vi "Mod_OFDM_Examine_Configure_OFDM_Frame.vi"(0 "Configuration in":variant=variant("Attribute Names"=variant(cluster{"Data Source Pool":string, "Modulator Source Pool":string, "OFDM SYMBOL POOL":string, "Symbol Table":string, "Sub Carrier Selection":string, "OFDM Frame":string, "FRAME Table":string, "Pulse Shaping":string} {"Data Source Pool"="Data Source ", "Modulator Source Pool"="Modulator Source Pool ", "OFDM SYMBOL POOL"="OFDM SYMBOL POOL", "Symbol Table"="Symbol Table", "Sub Carrier Selection"="Sub Carrier Selection", "OFDM Frame"="OFDM Frame", "FRAME Table"="FRAME Table", "Pulse Shaping"="Pulse Shaping"}), "Data Source "=variant(cluster{"mode (PN)":enum16{"PN", "pattern", "user"}, "PN sequence order (9)":i32, "Invert Output Bits":enum16{"No", "Yes"}, "Register Initial State":u32, "User base bit pattern":i8[], "base bit pattern (00001111)":enum16{"0", "1", "01", "0011", "00001111"}, "Reset to Initial State":enum16{"Every OFDM Frame", "Every OFDM Symbol", "Every Sub Carrier"}}[] [{"mode (PN)"=enum."PN", "PN sequence order (9)"=9, "Invert Output Bits"=enum."No", "Register Initial State"=3602873842, "User base bit pattern"=[], "base bit pattern (00001111)"=enum."00001111", "Reset to Initial State"=enum."Every OFDM Frame"}, {"mode (PN)"=enum."PN", "PN sequence order (9)"=9, "Invert Output Bits"=enum."No", "Register Initial State"=3602873842, "User base bit pattern"=[], "base bit pattern (00001111)"=enum."00001111", "Reset to Initial State"=enum."Every OFDM Frame"}, {"mode (PN)"=enum."PN", "PN sequence order (9)"=9, "Invert Output Bits"=enum."No", "Register Initial State"=3602873842, "User base bit pattern"=[], "base bit pattern (00001111)"=enum."00001111", "Reset to Initial State"=enum."Every OFDM Frame"}, {"mode (PN)"=enum."PN", "PN sequence order (9)"=9, "Invert Output Bits"=enum."No", "Register Initial State"=3602873842, "User base bit pattern"=[], "base bit pattern (00001111)"=enum."00001111", "Reset to Initial State"=enum."Every OFDM Frame"}]), "FRAME Table"=variant(string[][] []), "Modulator Source Pool "=variant(cluster{"M-QAM":enum16{"4", "16", "64", "256"}, "M-PSK":enum16{"2", "4", "8", "16", "32", "64", "128", "256"}, "Type of Modulation":enum16{"PSK", "QAM"}, "PSK":cluster{"differential PSK":enum16{"disable", "enable"}, "PSK type":enum16{"normal", "shifted", "offset"}}}[] [{"M-QAM"=enum."4", "M-PSK"=enum."2", "Type of Modulation"=enum."PSK", "PSK"={"differential PSK"=enum."disable", "PSK type"=enum."normal"}}, {"M-QAM"=enum."4", "M-PSK"=enum."2", "Type of Modulation"=enum."PSK", "PSK"={"differential PSK"=enum."disable", "PSK type"=enum."normal"}}, {"M-QAM"=enum."4", "M-PSK"=enum."2", "Type of Modulation"=enum."PSK", "PSK"={"differential PSK"=enum."disable", "PSK type"=enum."normal"}}, {"M-QAM"=enum."4", "M-PSK"=enum."2", "Type of Modulation"=enum."PSK", "PSK"={"differential PSK"=enum."disable", "PSK type"=enum."normal"}}]), "No_Name"=variant(cluster{"Sub Carrier Selection":cluster{"Sub Carrier":bool, "Data Source":u16, "Modulator":u16}[], "OFDM Parameters":cluster{"# of Sub Carrier":i32, "Length Of Cylic Prefix":i32}} {"Sub Carrier Selection"=[{"Sub Carrier"=TRUE, "Data Source"=0, "Modulator"=0}, {"Sub Carrier"=TRUE, "Data Source"=0, "Modulator"=0}, {"Sub Carrier"=TRUE, "Data Source"=0, "Modulator"=0}, {"Sub Carrier"=TRUE, "Data Source"=0, "Modulator"=0}, {"Sub Carrier"=TRUE, "Data Source"=0, "Modulator"=0}, {"Sub Carrier"=TRUE, "Data Source"=0, "Modulator"=0}, {"Sub Carrier"=TRUE, "Data Source"=0, "Modulator"=0}, {"Sub Carrier"=TRUE, "Data Source"=0, "Modulator"=0}, {"Sub Carrier"=TRUE, "Data Source"=0, "Modulator"=0}, {"Sub Carrier"=TRUE, "Data Source"=0, "Modulator"=0}, {"Sub Carrier"=TRUE, "Data Source"=0, "Modulator"=0}, {"Sub Carrier"=TRUE, "Data Source"=0, "Modulator"=0}, {"Sub Carrier"=TRUE, "Data Source"=0, "Modulator"=0}, {"Sub Carrier"=TRUE, "Data Source"=0, "Modulator"=0}, {"Sub Carrier"=TRUE, "Data Source"=0, "Modulator"=0}, {"Sub Carrier"=TRUE, "Data Source"=0, "Modulator"=0}, {"Sub Carrier"=TRUE, "Data Source"=0, "Modulator"=0}, {"Sub Carrier"=TRUE, "Data Source"=0, "Modulator"=0}, {"Sub Carrier"=TRUE, "Data Source"=0, "Modulator"=0}, {"Sub Carrier"=TRUE, "Data Source"=0, "Modulator"=0}, {"Sub Carrier"=TRUE, "Data Source"=0, "Modulator"=0}, {"Sub Carrier"=TRUE, "Data Source"=0, "Modulator"=0}, {"Sub Carrier"=TRUE, "Data Source"=0, "Modulator"=0}, {"Sub Carrier"=TRUE, "Data Source"=0, "Modulator"=0}, {"Sub Carrier"=TRUE, "Data Source"=0, "Modulator"=0}, {"Sub Carrier"=TRUE, "Data Source"=0, "Modulator"=0}, {"Sub Carrier"=TRUE, "Data Source"=0, "Modulator"=0}, {"Sub Carrier"=TRUE, "Data Source"=0, "Modulator"=0}, {"Sub Carrier"=TRUE, "Data Source"=0, "Modulator"=0}, {"Sub Carrier"=TRUE, "Data Source"=0, "Modulator"=0}, {"Sub Carrier"=TRUE, "Data Source"=0, "Modulator"=0}, {"Sub Carrier"=TRUE, "Data Source"=0, "Modulator"=0}, {"Sub Carrier"=TRUE, "Data Source"=0, "Modulator"=0}, {"Sub Carrier"=TRUE, "Data Source"=0, "Modulator"=0}, {"Sub Carrier"=TRUE, "Data Source"=0, "Modulator"=0}, {"Sub Carrier"=TRUE, "Data Source"=0, "Modulator"=0}, {"Sub Carrier"=TRUE, "Data Source"=0, "Modulator"=0}, {"Sub Carrier"=TRUE, "Data Source"=0, "Modulator"=0}, {"Sub Carrier"=TRUE, "Data Source"=0, "Modulator"=0}, {"Sub Carrier"=TRUE, "Data Source"=0, "Modulator"=0}, {"Sub Carrier"=TRUE, "Data Source"=0, "Modulator"=0}, {"Sub Carrier"=TRUE, "Data Source"=0, "Modulator"=0}, {"Sub Carrier"=TRUE, "Data Source"=0, "Modulator"=0}, {"Sub Carrier"=TRUE, "Data Source"=0, "Modulator"=0}, {"Sub Carrier"=TRUE, "Data Source"=0, "Modulator"=0}, {"Sub Carrier"=TRUE, "Data Source"=0, "Modulator"=0}, {"Sub Carrier"=TRUE, "Data Source"=0, "Modulator"=0}, {"Sub Carrier"=TRUE, "Data Source"=0, "Modulator"=2}, {"Sub Carrier"=TRUE, "Data Source"=0, "Modulator"=0}, {"Sub Carrier"=TRUE, "Data Source"=0, "Modulator"=0}, {"Sub Carrier"=TRUE, "Data Source"=0, "Modulator"=0}, {"Sub Carrier"=TRUE, "Data Source"=0, "Modulator"=0}, {"Sub Carrier"=TRUE, "Data Source"=0, "Modulator"=0}, {"Sub Carrier"=TRUE, "Data Source"=0, "Modulator"=0}, {"Sub Carrier"=TRUE, "Data Source"=0, "Modulator"=0}, {"Sub Carrier"=TRUE, "Data Source"=0, "Modulator"=0}, {"Sub Carrier"=TRUE, "Data Source"=0, "Modulator"=0}, {"Sub Carrier"=TRUE, "Data Source"=0, "Modulator"=0}, {"Sub Carrier"=TRUE, "Data Source"=0, "Modulator"=0}, {"Sub Carrier"=TRUE, "Data Source"=0, "Modulator"=0}, {"Sub Carrier"=TRUE, "Data Source"=0, "Modulator"=0}, {"Sub Carrier"=TRUE, "Data Source"=0, "Modulator"=0}, {"Sub Carrier"=TRUE, "Data Source"=0, "Modulator"=0}, {"Sub Carrier"=TRUE, "Data Source"=0, "Modulator"=0}], "OFDM Parameters"={"# of Sub Carrier"=64, "Length Of Cylic Prefix"=16}}), "OFDM Frame"=variant(cluster{"Symbol Name":string, "# of Symbols":i32}[] []), "OFDM SYMBOL POOL"=variant(string[] ["No_Name"]), "Pulse Shaping"=variant(cluster{"System Filter":cluster{"TX Filter":enum16{"none", "Raised Cosine", "Root Raised Cos"}, "Alpha":dbl, "filter length":i32}, "Modulation system parameters":cluster{"samples per symbol (16)":u32}, "symbol rate (Hz)":dbl} {"System Filter"={"TX Filter"=enum."Root Raised Cos", "Alpha"=0.5, "filter length"=8}, "Modulation system parameters"={"samples per symbol (16)"=16}, "symbol rate (Hz)"=100000.0}), "Sub Carrier Selection"=variant(cluster{"Sub Carrier Selection":cluster{"Sub Carrier":bool, "Data Source":u16, "Modulator":u16}[], "OFDM Parameters":cluster{"# of Sub Carrier":i32, "Length Of Cylic Prefix":i32}} {"Sub Carrier Selection"=array[10000 elements], "OFDM Parameters"={"# of Sub Carrier"=64, "Length Of Cylic Prefix"=16}}), "Symbol Table"=variant(string[][] [["-32", " ON", "   0", "   0"], ["-31", " ON", "   0", "   0"], ["-30", " ON", "   0", "   0"], ["-29", " ON", "   0", "   0"], ["-28", " ON", "   0", "   0"], ["-27", " ON", "   0", "   0"], ["-26", " ON", "   0", "   0"], ["-25", " ON", "   0", "   0"], ["-24", " ON", "   0", "   0"], ["-23", " ON", "   0", "   0"], ["-22", " ON", "   0", "   0"], ["-21", " ON", "   0", "   0"], ["-20", " ON", "   0", "   0"], ["-19", " ON", "   0", "   0"], ["-18", " ON", "   0", "   0"], ["-17", " ON", "   0", "   0"], ["-16", " ON", "   0", "   0"], ["-15", " ON", "   0", "   0"], ["-14", " ON", "   0", "   0"], ["-13", " ON", "   0", "   0"], ["-12", " ON", "   0", "   0"], ["-11", " ON", "   0", "   0"], ["-10", " ON", "   0", "   0"], ["-9", " ON", "   0", "   0"], ["-8", " ON", "   0", "   0"], ["-7", " ON", "   0", "   0"], ["-6", " ON", "   0", "   0"], ["-5", " ON", "   0", "   0"], ["-4", " ON", "   0", "   0"], ["-3", " ON", "   0", "   0"], ["-2", " ON", "   0", "   0"], ["-1", " ON", "   0", "   0"], ["0", " ON", "   0", "   0"], ["+1", " ON", "   0", "   0"], ["+2", " ON", "   0", "   0"], ["+3", " ON", "   0", "   0"], ["+4", " ON", "   0", "   0"], ["+5", " ON", "   0", "   0"], ["+6", " ON", "   0", "   0"], ["+7", " ON", "   0", "   0"], ["+8", " ON", "   0", "   0"], ["+9", " ON", "   0", "   0"], ["+10", " ON", "   0", "   0"], ["+11", " ON", "   0", "   0"], ["+12", " ON", "   0", "   0"], ["+13", " ON", "   0", "   0"], ["+14", " ON", "   0", "   0"], ["+15", " ON", "   0", "   2"], ["+16", " ON", "   0", "   0"], ["+17", " ON", "   0", "   0"], ["+18", " ON", "   0", "   0"], ["+19", " ON", "   0", "   0"], ["+20", " ON", "   0", "   0"], ["+21", " ON", "   0", "   0"], ["+22", " ON", "   0", "   0"], ["+23", " ON", "   0", "   0"], ["+24", " ON", "   0", "   0"], ["+25", " ON", "   0", "   0"], ["+26", " ON", "   0", "   0"], ["+27", " ON", "   0", "   0"], ["+28", " ON", "   0", "   0"], ["+29", " ON", "   0", "   0"], ["+30", " ON", "   0", "   0"], ["+31", " ON", "   0", "   0"]])), 5 "Configure OFDM Frame":T1={"Symbol Pool"=0, "Add"=FALSE, "Delete"=FALSE, "# of Symbols"=1} {"# of Symbols" min=1; "Symbol Pool" items=["IEEE 802.11a First Symbol of Frame", "IEEE 802.11a Frame (BPSK)", "IEEE 802.11a Frame (QPSK)", "IEEE 802.11a Frame (16QAM)", "IEEE 802.11a Frame (64QAM)", "No_Name"]}, 11 "error in":errorcluster) -> (4 "Configuration out":variant=variant("Attribute Names"=variant(cluster{"Data Source Pool":string, "Modulator Source Pool":string, "OFDM SYMBOL POOL":string, "Symbol Table":string, "Sub Carrier Selection":string, "OFDM Frame":string, "FRAME Table":string, "Pulse Shaping":string} {"Data Source Pool"="Data Source ", "Modulator Source Pool"="Modulator Source Pool ", "OFDM SYMBOL POOL"="OFDM SYMBOL POOL", "Symbol Table"="Symbol Table", "Sub Carrier Selection"="Sub Carrier Selection", "OFDM Frame"="OFDM Frame", "FRAME Table"="FRAME Table", "Pulse Shaping"="Pulse Shaping"}), "Data Source "=variant(cluster{"mode (PN)":enum16{"PN", "pattern", "user"}, "PN sequence order (9)":i32, "Invert Output Bits":enum16{"No", "Yes"}, "Register Initial State":u32, "User base bit pattern":i8[], "base bit pattern (00001111)":enum16{"0", "1", "01", "0011", "00001111"}, "Reset to Initial State":enum16{"Every OFDM Frame", "Every OFDM Symbol", "Every Sub Carrier"}}[] [{"mode (PN)"=enum."PN", "PN sequence order (9)"=9, "Invert Output Bits"=enum."No", "Register Initial State"=3602873842, "User base bit pattern"=[], "base bit pattern (00001111)"=enum."00001111", "Reset to Initial State"=enum."Every OFDM Frame"}, {"mode (PN)"=enum."PN", "PN sequence order (9)"=9, "Invert Output Bits"=enum."No", "Register Initial State"=3602873842, "User base bit pattern"=[], "base bit pattern (00001111)"=enum."00001111", "Reset to Initial State"=enum."Every OFDM Frame"}, {"mode (PN)"=enum."PN", "PN sequence order (9)"=9, "Invert Output Bits"=enum."No", "Register Initial State"=3602873842, "User base bit pattern"=[], "base bit pattern (00001111)"=enum."00001111", "Reset to Initial State"=enum."Every OFDM Frame"}, {"mode (PN)"=enum."PN", "PN sequence order (9)"=9, "Invert Output Bits"=enum."No", "Register Initial State"=3602873842, "User base bit pattern"=[], "base bit pattern (00001111)"=enum."00001111", "Reset to Initial State"=enum."Every OFDM Frame"}]), "FRAME Table"=variant(string[][] []), "Modulator Source Pool "=variant(cluster{"M-QAM":enum16{"4", "16", "64", "256"}, "M-PSK":enum16{"2", "4", "8", "16", "32", "64", "128", "256"}, "Type of Modulation":enum16{"PSK", "QAM"}, "PSK":cluster{"differential PSK":enum16{"disable", "enable"}, "PSK type":enum16{"normal", "shifted", "offset"}}}[] [{"M-QAM"=enum."4", "M-PSK"=enum."2", "Type of Modulation"=enum."PSK", "PSK"={"differential PSK"=enum."disable", "PSK type"=enum."normal"}}, {"M-QAM"=enum."4", "M-PSK"=enum."2", "Type of Modulation"=enum."PSK", "PSK"={"differential PSK"=enum."disable", "PSK type"=enum."normal"}}, {"M-QAM"=enum."4", "M-PSK"=enum."2", "Type of Modulation"=enum."PSK", "PSK"={"differential PSK"=enum."disable", "PSK type"=enum."normal"}}, {"M-QAM"=enum."4", "M-PSK"=enum."2", "Type of Modulation"=enum."PSK", "PSK"={"differential PSK"=enum."disable", "PSK type"=enum."normal"}}]), "No_Name"=variant(cluster{"Sub Carrier Selection":cluster{"Sub Carrier":bool, "Data Source":u16, "Modulator":u16}[], "OFDM Parameters":cluster{"# of Sub Carrier":i32, "Length Of Cylic Prefix":i32}} {"Sub Carrier Selection"=[{"Sub Carrier"=TRUE, "Data Source"=0, "Modulator"=0}, {"Sub Carrier"=TRUE, "Data Source"=0, "Modulator"=0}, {"Sub Carrier"=TRUE, "Data Source"=0, "Modulator"=0}, {"Sub Carrier"=TRUE, "Data Source"=0, "Modulator"=0}, {"Sub Carrier"=TRUE, "Data Source"=0, "Modulator"=0}, {"Sub Carrier"=TRUE, "Data Source"=0, "Modulator"=0}, {"Sub Carrier"=TRUE, "Data Source"=0, "Modulator"=0}, {"Sub Carrier"=TRUE, "Data Source"=0, "Modulator"=0}, {"Sub Carrier"=TRUE, "Data Source"=0, "Modulator"=0}, {"Sub Carrier"=TRUE, "Data Source"=0, "Modulator"=0}, {"Sub Carrier"=TRUE, "Data Source"=0, "Modulator"=0}, {"Sub Carrier"=TRUE, "Data Source"=0, "Modulator"=0}, {"Sub Carrier"=TRUE, "Data Source"=0, "Modulator"=0}, {"Sub Carrier"=TRUE, "Data Source"=0, "Modulator"=0}, {"Sub Carrier"=TRUE, "Data Source"=0, "Modulator"=0}, {"Sub Carrier"=TRUE, "Data Source"=0, "Modulator"=0}, {"Sub Carrier"=TRUE, "Data Source"=0, "Modulator"=0}, {"Sub Carrier"=TRUE, "Data Source"=0, "Modulator"=0}, {"Sub Carrier"=TRUE, "Data Source"=0, "Modulator"=0}, {"Sub Carrier"=TRUE, "Data Source"=0, "Modulator"=0}, {"Sub Carrier"=TRUE, "Data Source"=0, "Modulator"=0}, {"Sub Carrier"=TRUE, "Data Source"=0, "Modulator"=0}, {"Sub Carrier"=TRUE, "Data Source"=0, "Modulator"=0}, {"Sub Carrier"=TRUE, "Data Source"=0, "Modulator"=0}, {"Sub Carrier"=TRUE, "Data Source"=0, "Modulator"=0}, {"Sub Carrier"=TRUE, "Data Source"=0, "Modulator"=0}, {"Sub Carrier"=TRUE, "Data Source"=0, "Modulator"=0}, {"Sub Carrier"=TRUE, "Data Source"=0, "Modulator"=0}, {"Sub Carrier"=TRUE, "Data Source"=0, "Modulator"=0}, {"Sub Carrier"=TRUE, "Data Source"=0, "Modulator"=0}, {"Sub Carrier"=TRUE, "Data Source"=0, "Modulator"=0}, {"Sub Carrier"=TRUE, "Data Source"=0, "Modulator"=0}, {"Sub Carrier"=TRUE, "Data Source"=0, "Modulator"=0}, {"Sub Carrier"=TRUE, "Data Source"=0, "Modulator"=0}, {"Sub Carrier"=TRUE, "Data Source"=0, "Modulator"=0}, {"Sub Carrier"=TRUE, "Data Source"=0, "Modulator"=0}, {"Sub Carrier"=TRUE, "Data Source"=0, "Modulator"=0}, {"Sub Carrier"=TRUE, "Data Source"=0, "Modulator"=0}, {"Sub Carrier"=TRUE, "Data Source"=0, "Modulator"=0}, {"Sub Carrier"=TRUE, "Data Source"=0, "Modulator"=0}, {"Sub Carrier"=TRUE, "Data Source"=0, "Modulator"=0}, {"Sub Carrier"=TRUE, "Data Source"=0, "Modulator"=0}, {"Sub Carrier"=TRUE, "Data Source"=0, "Modulator"=0}, {"Sub Carrier"=TRUE, "Data Source"=0, "Modulator"=0}, {"Sub Carrier"=TRUE, "Data Source"=0, "Modulator"=0}, {"Sub Carrier"=TRUE, "Data Source"=0, "Modulator"=0}, {"Sub Carrier"=TRUE, "Data Source"=0, "Modulator"=0}, {"Sub Carrier"=TRUE, "Data Source"=0, "Modulator"=2}, {"Sub Carrier"=TRUE, "Data Source"=0, "Modulator"=0}, {"Sub Carrier"=TRUE, "Data Source"=0, "Modulator"=0}, {"Sub Carrier"=TRUE, "Data Source"=0, "Modulator"=0}, {"Sub Carrier"=TRUE, "Data Source"=0, "Modulator"=0}, {"Sub Carrier"=TRUE, "Data Source"=0, "Modulator"=0}, {"Sub Carrier"=TRUE, "Data Source"=0, "Modulator"=0}, {"Sub Carrier"=TRUE, "Data Source"=0, "Modulator"=0}, {"Sub Carrier"=TRUE, "Data Source"=0, "Modulator"=0}, {"Sub Carrier"=TRUE, "Data Source"=0, "Modulator"=0}, {"Sub Carrier"=TRUE, "Data Source"=0, "Modulator"=0}, {"Sub Carrier"=TRUE, "Data Source"=0, "Modulator"=0}, {"Sub Carrier"=TRUE, "Data Source"=0, "Modulator"=0}, {"Sub Carrier"=TRUE, "Data Source"=0, "Modulator"=0}, {"Sub Carrier"=TRUE, "Data Source"=0, "Modulator"=0}, {"Sub Carrier"=TRUE, "Data Source"=0, "Modulator"=0}, {"Sub Carrier"=TRUE, "Data Source"=0, "Modulator"=0}], "OFDM Parameters"={"# of Sub Carrier"=64, "Length Of Cylic Prefix"=16}}), "OFDM Frame"=variant(cluster{"Symbol Name":string, "# of Symbols":i32}[] []), "OFDM SYMBOL POOL"=variant(string[] ["No_Name"]), "Pulse Shaping"=variant(cluster{"System Filter":cluster{"TX Filter":enum16{"none", "Raised Cosine", "Root Raised Cos"}, "Alpha":dbl, "filter length":i32}, "Modulation system parameters":cluster{"samples per symbol (16)":u32}, "symbol rate (Hz)":dbl} {"System Filter"={"TX Filter"=enum."Root Raised Cos", "Alpha"=0.5, "filter length"=8}, "Modulation system parameters"={"samples per symbol (16)"=16}, "symbol rate (Hz)"=100000.0}), "Sub Carrier Selection"=variant(cluster{"Sub Carrier Selection":cluster{"Sub Carrier":bool, "Data Source":u16, "Modulator":u16}[], "OFDM Parameters":cluster{"# of Sub Carrier":i32, "Length Of Cylic Prefix":i32}} {"Sub Carrier Selection"=array[10000 elements], "OFDM Parameters"={"# of Sub Carrier"=0, "Length Of Cylic Prefix"=0}}), "Symbol Table"=variant(string[][] [])), 15 "error out":errorcluster)   [LabVIEW 2010]
doc: "Configures OFDM Frame that is to be generated. A Frame is defined as a certain time span that is filled with OFDM Symbols. Frame is the highest layer of organization within the time structure of the signal to generate."
uses:
  Polymorphic_Sub_VI's/Mod_OFDM_Get_FRAME_Table.vi
panel:
  out "Symbol Table":string[][](table)
  out "OFDM Symbol":string
  out "Frame Table":string[][](table)
  in  "Cancel Operation":bool
  in  "Apply Settings":bool
  # "Note:\nAdds/Deletes\nOFDM symbols\nfrom the selected \nrow"
  # "Sub_\nCarrier"
  # "Data\nSource"
  # "Modulator\nSource"
  # "Status"
  # "# of\nSymbols"
  # "Total\nSymbols"
  # "OFDM Symbol"
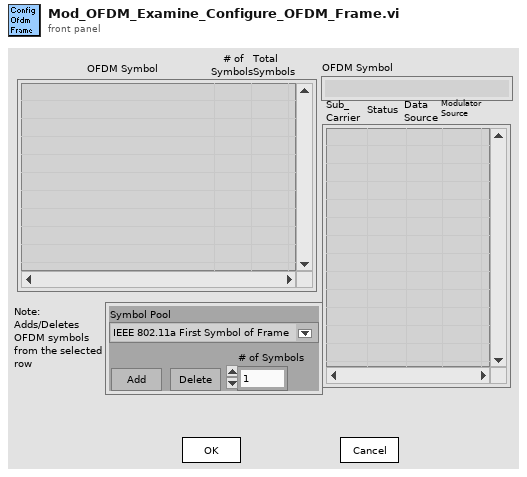
[diagram p1: front panel]
types:
  T1 = cluster{"Symbol Pool":u16, "Add":bool, "Delete":bool, "# of Symbols":u32}
  T2 = typedef "LVRowAndColumnTypeDef.ctl" = cluster{"Row":i32, "Column":i32}
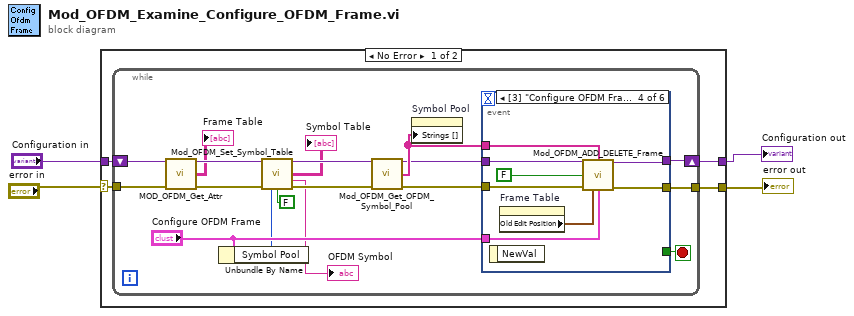
[diagram p0: block diagram]
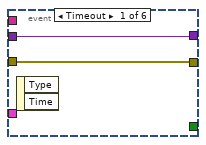
[diagram p2: hidden frame]
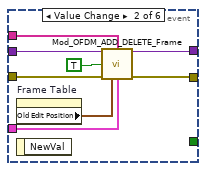
[diagram p3: hidden frame]
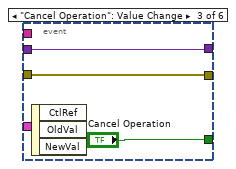
[diagram p4: hidden frame]
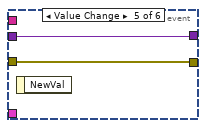
[diagram p5: hidden frame]
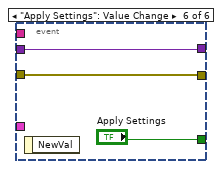
[diagram p6: hidden frame]
diagram:
  n1 = case shown="No Error" "error in" {
    selector: "error in" -> [w5 w53]
    tunnel: "Configuration in" -> [w8 _]
    tunnel: [w7 _] -> w3
    tunnel: [w6 w53] -> w2
    frame No Error {
      n2 = while {
        shift-right: [w26] -> w7
        shift-left: w8 -> [w24]
        tunnel: w5 -> [w23]
        tunnel: [w22] -> w6
        stop <- w25 stop-if-true
        n3 = call-poly "MOD_OFDM_Get_Attr.vi"("Configuration in"=w24, "error in"=w23) -> ("Configuration out"=w18:variant, "FRAME Table"=→"Frame Table":string[][], "error out"=w16:errorcluster)  [unwired: 11 in]
        n4 = Unbundle By Name("Configure OFDM Frame") -> ("Symbol Pool"=w11:u16)
        n5 = call "Mod_OFDM_Set_Symbol_Table.vi"("Configuration in"=w18, "error in"=w16, "Symbol Pool"=w11, "Configure/\nRetrieve"=FALSE ("Configure/\nRetrieve")) -> ("Configuration out"=w17:variant, "Symbol Table"=→"Symbol Table":string[][], "Current OFDM Symbol Name(O/P)"=→"OFDM Symbol":string, "error out"=w15:errorcluster)  [unwired: 7 in, 1 out]
        n6 = call-poly "Mod_OFDM_Get_OFDM_Symbol_Pool.vi"("Configuration in"=w17, "error in"=w15) -> ("Configuration out"=w19:variant, "Symbol Pool"=w20:string[], "error out"=w21:errorcluster)  [unwired: 8 in, 3 out]
        n7 = property on="Symbol Pool" class="Ring (strict)"("Strings []"=w20) -> ()  [unwired: 2 in, 2 out]
        n8 = event shown="[3] \"Configure OFDM Frame .Delete\": Value Change" {
          selector: _ -> [_ _ _ _ _ _]
          dyn-events: _ -> [_ _ _ _ _ _]
          timeout: _ -> [_ _ _ _ _ _]
          tunnel: w19 -> [w28 w36 w38 w47 w49 w52]
          tunnel: [w28 w32 w38 w42 w49 w52] -> w26
          tunnel: w20 -> [_ w33 _ w45 _ _]
          tunnel: [_ _ "Cancel Operation" _ _ "Apply Settings"] -> w25
          tunnel: "Configure OFDM Frame" -> [_ w34 _ w44 _ _]
          tunnel: w21 -> [w27 w35 w37 w46 w48 w50]
          tunnel: [w27 w31 w37 w43 w48 w50] -> w22
          event Timeout {
            n9 = event-data() -> ()  [unwired: 1 in, 2 out]
          }
          event "Configure OFDM Frame.Add": Value Change {
            n10 = property on="Frame Table" class="Tbl (strict)"() -> ("Old Edit Position"=w29:T2)  [unwired: 2 in, 2 out]
            n11 = event-data() -> ()  [unwired: 1 in, 1 out]
            n12 = call "Mod_OFDM_ADD_DELETE_Frame.vi"("Configuration in"=w36, "OFDM SYmbol Pool"=w33, "Add/delete"=TRUE, "error in"=w35, "Edit Position"=w29, "Config OFDM Frame"=w34) -> ("Configuration out"=w32:variant, "error out"=w31:errorcluster)  [unwired: 8 in]
          }
          event "Cancel Operation": Value Change {
            n13 = event-data() -> ()  [unwired: 1 in, 3 out]
          }
          event "Configure OFDM Frame.Delete": Value Change {
            n14 = event-data() -> ()  [unwired: 1 in, 1 out]
            n15 = property on="Frame Table" class="Tbl (strict)"() -> ("Old Edit Position"=w40:T2)  [unwired: 2 in, 2 out]
            n16 = call "Mod_OFDM_ADD_DELETE_Frame.vi"("Configuration in"=w47, "OFDM SYmbol Pool"=w45, "Add/delete"=FALSE, "error in"=w46, "Edit Position"=w40, "Config OFDM Frame"=w44) -> ("Configuration out"=w42:variant, "error out"=w43:errorcluster)  [unwired: 8 in]
          }
          event "Configure OFDM Frame.Symbol Pool", "Configure OFDM Frame.# of Symbols": Value Change {
            n17 = event-data() -> ()  [unwired: 1 in, 1 out]
          }
          event "Apply Settings": Value Change {
            n18 = event-data() -> ()  [unwired: 1 in, 1 out]
          }
        }
      }
    }
    frame Error {
    }
  }
  "Configuration out" <- w3
  "error out" <- w2
